vi "PAN_ObtainCmdID.vi"(5 "send cmdid":bool, 7 "source":string, 10 "resp in":string, 11 "Database RefNum in":T1) -> (2 "resp out":string)   [LabVIEW 2016]
uses:
  Modules/DBSHAND/private/vis/DatabaseHand_RefNum.ctl
  Modules/DBSHAND/private/vis/DatabaseHand_Element_Get(string).vi
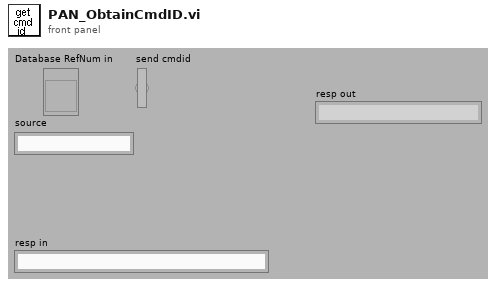
[diagram p1: front panel]
types:
  T1 = typedef "DatabaseHand_RefNum.ctl" = refnum<vi>
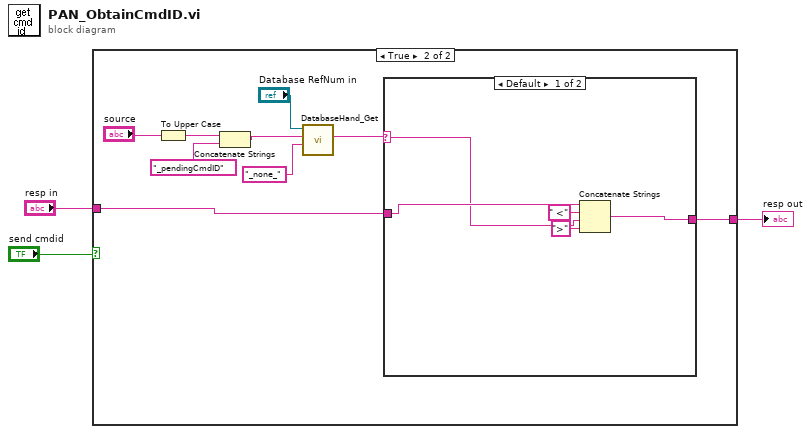
[diagram p0: block diagram]
diagram:
  n1 = case shown="True" "send cmdid" {
    tunnel: "resp in" -> [w4 w8]
    tunnel: [w4 w7] -> w2
    frame False {
    }
    frame True {
      n2 = To Upper Case(1:"source") -> (0:w10:string)
      n3 = Concatenate Strings(w10, "_pendingCmdID" ("name")) -> (w6:string)
      n4 = call-poly "DatabaseHand_Get.vi"("default value"="_none_", "name"=w6, "Database RefNum in"="Database RefNum in") -> ("value"=w9:string)  [unwired: 2 in, 6 out]
      n5 = case shown="Default" w9 {
        selector: w9 -> [w15 _]
        tunnel: w8 -> [w17 w19]
        tunnel: [w18 w19] -> w7
        frame Default {
          n6 = Concatenate Strings(w17, " <" ("string"), w15, ">" ("string")) -> (w18:string)
        }
        frame "_none_" {
        }
      }
    }
  }
  "resp out" <- w2
